vi "Channels Array to Channels String.vi"(8 "error in (no error)":errorcluster, 10 "Channel(s) Array":T1[](array[typedef]), 11 "PXIe5105 in":refnum<class "PXIe5105.lvclass">) -> (0 "error out":errorcluster, 2 "Channels String":string, 3 "PXIe5105 out":refnum<class "PXIe5105.lvclass">)   [LabVIEW 2018, in "PXIe5105.lvlib" / "PXIe5105.lvclass"]
uses:
  PXIe5105.lvclass
  PPLs/Oscilloscope/Parent/Oscilloscope.lvlibp/Custom Controls/Analog Channels.ctl
  PPLs/Oscilloscope/Parent/Oscilloscope.lvlibp
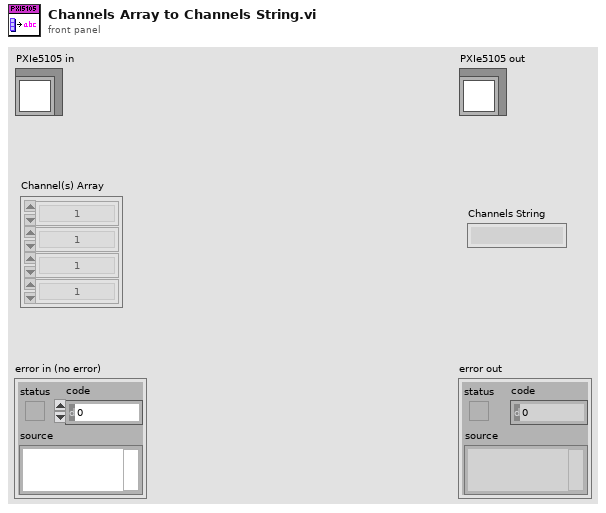
[diagram p1: front panel]
types:
  T1 = typedef "Oscilloscope.lvlibp/Analog Channels.ctl" = enum16{"1", "2", "3", "4", "5", "6", "7", "8", "9", "10", "11", "12", "13", "14", "15", "16"}
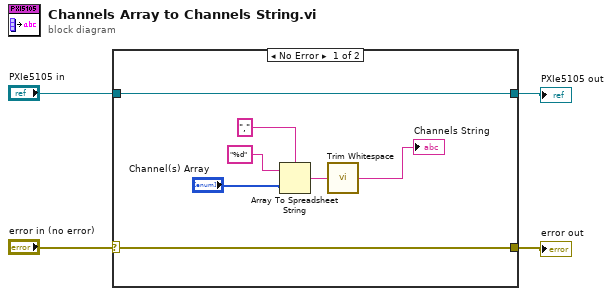
[diagram p0: block diagram]
diagram:
  n1 = case shown="No Error" "error in (no error)" {
    selector: "error in (no error)" -> [w10 w13]
    tunnel: [w10 w13] -> w3
    tunnel: [w11 w12] -> w1
    tunnel: "PXIe5105 in" -> [w11 w12]
    frame No Error {
      n2 = Array To Spreadsheet String(delimiter (Tab)=",", array="Channel(s) Array", 3:"%d" ("format string")) -> (spreadsheet string=w6:string)
      n3 = call <vilib>:"Trim Whitespace.vi"("string"=w6) -> ("trimmed string"=→"Channels String":string)  [unwired: 1 in]
    }
    frame Error {
    }
  }
  "error out" <- w3
  "PXIe5105 out" <- w1
